vi "Aim via Angle.vi"(2 "Initial Speed(in/s)":dbl=471.0, 3 "Vision Distance(in)":dbl) -> (0 "error out":errorcluster, 1 "Angle(degrees)":dbl)   [LabVIEW 2015]
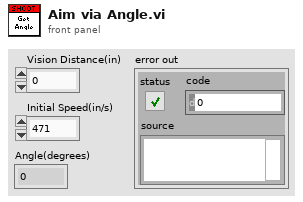
[diagram p1: front panel]
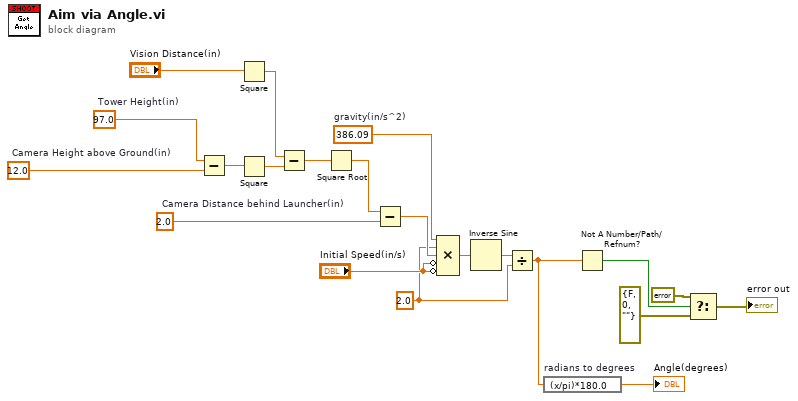
[diagram p0: block diagram]
diagram:
  w7 = 2.0 ("value")
  w20 = 386.09  # gravity(in/s^2)
  w17 = 2.0  # Camera Distance behind Launcher(in)
  w15 = 12.0  # Camera Height above Ground(in)
  w16 = 97.0  # Tower Height(in)
  n1 = Subtract(x=w16, y=w15) -> (x-y=w18:dbl)
  n2 = Square(x="Vision Distance(in)") -> (x^2=w11:dbl)
  n3 = Square(x=w18) -> (x^2=w12:dbl)
  n4 = Subtract(x=w11, y=w12) -> (x-y=w13:dbl)
  n5 = Square Root(x=w13) -> (sqrt(x)=w10:dbl)
  n6 = Subtract(x=w10, y=w17) -> (x-y=w9:dbl)
  n7 = Compound Arithmetic op=MULTIPLY(w20, w7, w9, invert "Initial Speed(in/s)", invert "Initial Speed(in/s)") -> (w19:dbl)
  n8 = Inverse Sine(1:w19) -> (0:w21:dbl)
  n9 = Divide(x=w21, y=w7) -> (x/y=w3:dbl)
  n10 = expression code="(x/pi)*180.0" "radians to degrees"(w3) -> (→"Angle(degrees)":dbl)
  n11 = Not A Number/Path/Refnum?(number/path/refnum=w3) -> (NaN/Path/Refnum?=w6:bool)
  n12 = Select(t=errorcluster {"status"=TRUE, "code"=9001, "source"="Speed not fast enough to score ball at this distance!"} ("error constant"), s=w6, f=errorcluster {"status"=FALSE, "code"=0, "source"=""}) -> (s? t:f=→"error out":errorcluster)
